vi "Action Set Fault Mode.vi"(5 "Retry Attempts (0)":i32 min=0, 7 "Fast Comms (F)":bool, 8 "error in (no error)":errorcluster, 11 "VISA resource name":refnum<visa-resource-name>) -> (0 "error out":errorcluster, 3 "VISA resource name out":refnum<visa-resource-name>)   [LabVIEW 2020, in "ChromTech Series I Drivers.lvlib"]
uses:
  <instrlib>/RxnRover/ChromtechSeriesIDriver/ChromTech Series I Drivers.lvlib
panel:
  out "Response":string
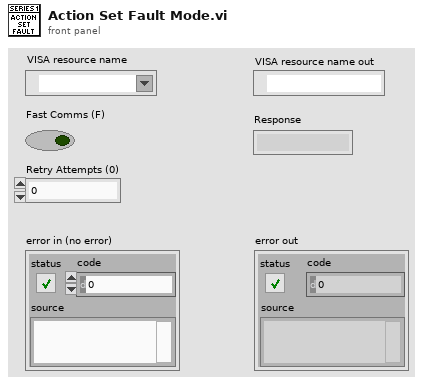
[diagram p1: front panel]
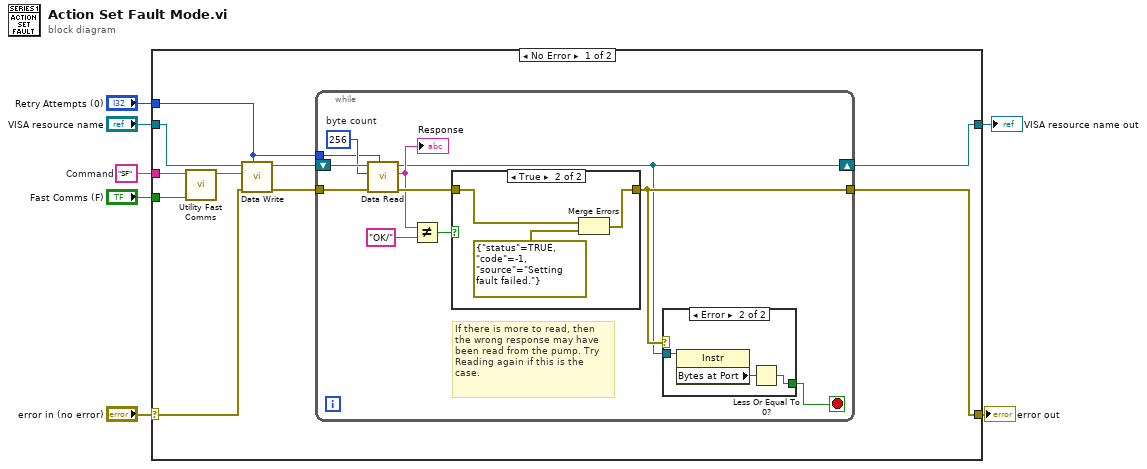
[diagram p0: block diagram]
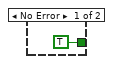
[diagram p2: hidden frame]
diagram:
  w3 = "SF"  # Command
  n1 = case shown="No Error" "error in (no error)" {
    selector: "error in (no error)" -> [w11 w37]
    tunnel: [w10 w37] -> w6
    tunnel: "VISA resource name" -> [w14 w38]
    tunnel: [w8 w38] -> w4
    tunnel: w3 -> [w13 _]
    tunnel: "Fast Comms (F)" -> [w12 _]
    tunnel: "Retry Attempts (0)" -> [w9 _]
    frame No Error {
      n2 = call <instrlib>:"Utility Fast Comms.vi"("Fast Comms"=w12, "Command"=w13) -> ("Fast Command"=w16:string)  [unwired: 9 in]
      n3 = call <instrlib>:"Data Write.vi"("Retry Attempts (0)"=w9, "error in (no error)"=w11, "Command"=w16, "VISA Refnum in"=w14) -> ("error out"=w15:errorcluster, "VISA Refnum out"=w17:refnum<visa-resource-name>)  [unwired: 6 in]
      n4 = while {
        tunnel: w9 -> [w21]
        shift-right: [w19] -> w8
        shift-left: w17 -> [w28]
        tunnel: w15 -> [w24]
        tunnel: [w20] -> w10
        stop <- w18 stop-if-true
        w27 = u32 256  # byte count
        # "If there is more to read, then\nthe wrong response may have\nbeen read from the pump. Try\nReading again if this is the\ncase."
        n5 = call <instrlib>:"Data Read.vi"("Retry Attempts (0)"=w21, "error in (no error)"=w24, "Bytes to read"=w27, "VISA Refnum in"=w28) -> ("error out"=w23:errorcluster, "read buffer"=w22:string, "VISA Refnum out"=w19:refnum<visa-resource-name>)  [unwired: 5 in]
        "Response" <- w22
        n6 = Not Equal?(x=w22, y="OK/") -> (x != y?=w25:bool)
        n7 = case shown="True" w25 {
          tunnel: [w33 w35] -> w20
          tunnel: w23 -> [w33 w34]
          frame False {
          }
          frame True {
            n8 = Merge Errors(w34, errorcluster {"status"=TRUE, "code"=-1, "source"="Setting fault failed."} ("error out")) -> (w35:errorcluster)
          }
        }
        n9 = case shown="Error" w20 {
          tunnel: w19 -> [_ w32]
          tunnel: [TRUE w30] -> w18
          frame No Error {
          }
          frame Error {
            n10 = property class="Instr"(reference=w32) -> ("Bytes at Port"=w31:u32)  [unwired: 1 in, 2 out]
            n11 = Less Or Equal To 0?(x=w31) -> (x <= 0?=w30:bool)
          }
        }
      }
    }
    frame Error {
    }
  }
  "error out" <- w6
  "VISA resource name out" <- w4
